vi "Launch Dialog Box.vi"(8 "error in (no error)":errorcluster, 10 "DialogBox":refnum<class "IDialogBox.lvclass">, 11 "IViewable In":refnum<class "IViewable.lvclass">) -> (0 "error out":errorcluster, 3 "IViewable Out":refnum<class "IViewable.lvclass">)   [LabVIEW 2015, in "IViewable.lvlib" / "IViewable.lvclass"]
doc: "<License>\nCopyright © 2017 Composed Systems, LLC | All rights reserved\nwww.composed.io\n\nAuthor: Ethan Stern <ethan.stern@composed.io>\n\nThis software is provided \"AS IS\" WITHOUT WARRANTIES, either express or implied, AND IS FOR EDUCATIONAL PURPOSES ONLY.\n</License>"
uses:
  IViewable.lvclass
  IDialogBox/IDialogBox/IDialogBox.lvclass
  IViewable.lvclass/IViewable.ctl
  <vilib>/ActorFramework/Message Enqueuer/Message Enqueuer.lvclass/Message Enqueuer.ctl
  <vilib>/ActorFramework/Message Enqueuer/Enqueue.vi
  <vilib>/ActorFramework/Message Priority Queue/Priority Enqueue.vi
  <vilib>/ActorFramework/Stop Msg/Stop Msg.lvclass
  <vilib>/ActorFramework/Actor/Actor.lvclass
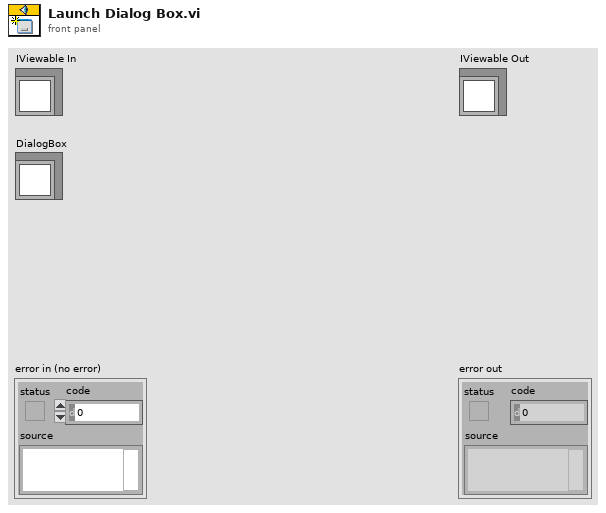
[diagram p1: front panel]
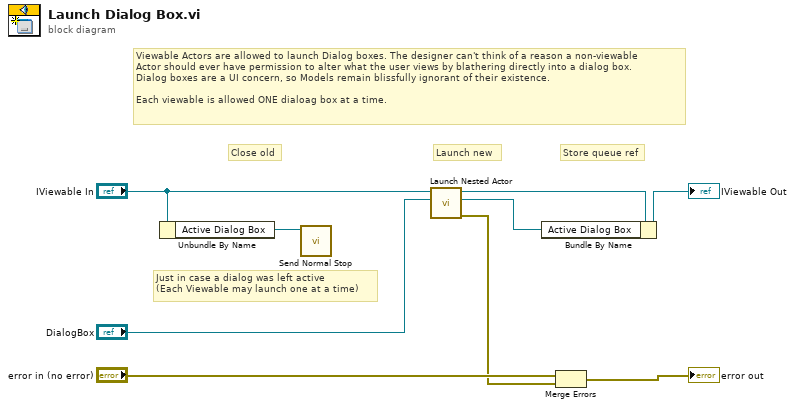
[diagram p0: block diagram]
diagram:
  # "Viewable Actors are allowed to launch Dialog boxes. The designer can't think of a reason a non-viewable\nActor should ever have permission to alter what the user views by blathering directly into a dialog box.\nDialog boxes are a UI concern, so Models remain blissfully ignorant of their existence.\n\nEach viewable is allowed ONE dialoag box at a time."
  # "Store queue ref"
  # "Launch new"
  # "Close old"
  # "Just in case a dialog was left active\n(Each Viewable may launch one at a time)"
  n1 = Unbundle By Name("IViewable In") -> ("Active Dialog Box"=w6:refnum<class "Message Enqueuer.lvclass">)
  n2 = call <vilib>:"Send Normal Stop.vi"("Message Enqueuer"=w6) -> ()  [unwired: 10 in, 1 out]
  n3 = call <vilib>:"Launch Nested Actor.vi"("Nested Actor"="DialogBox", "Caller Actor in"="IViewable In") -> ("error out"=w1:errorcluster, "Nested Actor's Enqueuer"=w3:refnum<class "Message Enqueuer.lvclass">, "Caller Actor out"=w8:refnum<class "IViewable.lvclass">)  [unwired: 7 in]
  n4 = Bundle By Name(cluster=w8, "Active Dialog Box"=w3) -> (→"IViewable Out":refnum<class "IViewable.lvclass">)
  n5 = Merge Errors("error in (no error)", w1) -> (→"error out":errorcluster)
